vi "Manipulator Get Sensor XYZ.vi"(8 "error in (no error)":errorcluster, 11 "VISA resource in":refnum<visa-resource-name>="COM1") -> (0 "error out":errorcluster, 2 "output cluster":cluster{"X":i32, "Y":i32, "Z":i32, "A":i32}, 3 "VISA resource out":refnum<visa-resource-name>)   [LabVIEW 2012, in "Scientifica Manipulator Daemon.lvlib"]
uses:
  Scientifica Manipulator Daemon.lvlib
panel:
  in  "Dummy Cluster":cluster{"X":i32, "Y":i32, "Z":i32, "A":i32}
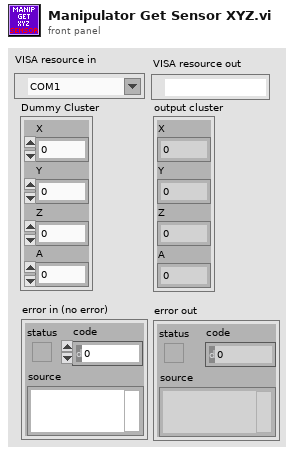
[diagram p1: front panel]
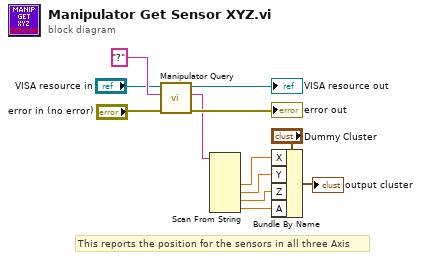
[diagram p0: block diagram]
diagram:
  # "This reports the position for the sensors in all three Axis"
  n1 = call "Manipulator Query.vi"("error in (no error)"="error in (no error)", "Command"="?", "VISA resource in"="VISA resource in") -> ("error out"=→"error out":errorcluster, "Response"=w6:string, "VISA resource out"=→"VISA resource out":refnum<visa-resource-name>)  [unwired: 5 in, 1 out]
  n2 = Scan From String(input string=w6) -> (output 1=w4:dbl, output 2=w3:dbl, output 3=w2:dbl, output 4=w1:dbl)  [unwired: 7 in, 3 out]
  n3 = Bundle By Name(cluster="Dummy Cluster", "X"=w4, "Y"=w3, "Z"=w2, "A"=w1) -> (→"output cluster":cluster{"X":i32, "Y":i32, "Z":i32, "A":i32})
